vi "FestoCPX.Init.vi"(8 "error in (no error)":errorcluster, 11 "Data in":T1={"Status"={"State"=enum."First", "Conn"=refnum, "TS"=timestamp(0 s since 1904-01-01)}, "Sets"={"IP"="", "Timeout_ms"=1, "ReconnectPeriod_s"=0, "Config.DI"=[], "Config.DO"=[]}}) -> (0 "error out":errorcluster, 3 "Data out":T1={"Status"={"State"=enum."First", "Conn"=refnum, "TS"=timestamp(0 s since 1904-01-01)}, "Sets"={"IP"="", "Timeout_ms"=1, "ReconnectPeriod_s"=0, "Config.DI"=[], "Config.DO"=[]}})   [LabVIEW 2015]
uses:
  FestoCPX.Data.ctl
  FestoCPX.Data.Status.ctl
  FestoCPX.State.ctl
  FestoCPX.Data.Sets.ctl
  FestoCPX.DI.Sets.ctl
  FestoCPX.DI.ctl
  FestoCPX.DO.Sets.ctl
  FestoCPX.DO.ctl
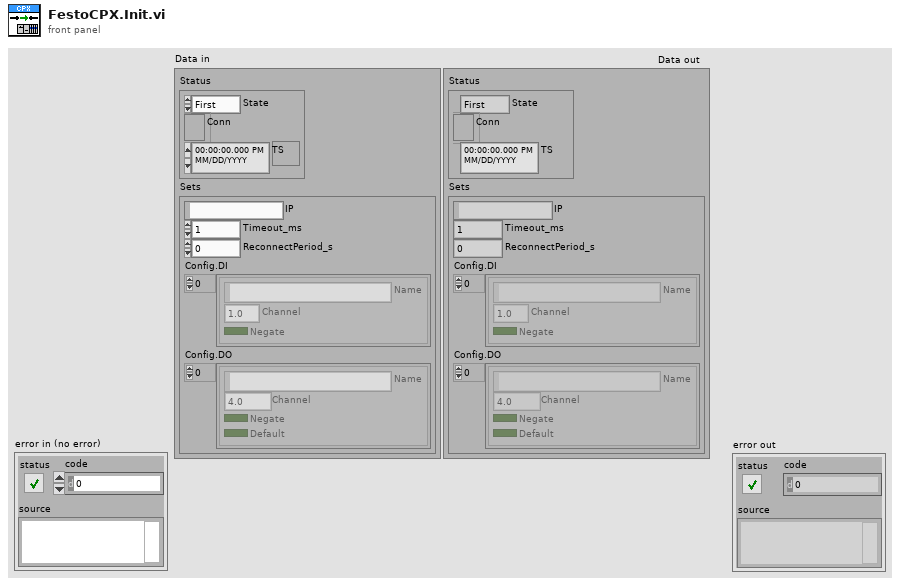
[diagram p1: front panel]
types:
  T1 = typedef "FestoCPX.Data.ctl" = cluster{"Status":T2, "Sets":T4}
  T2 = typedef "FestoCPX.Data.Status.ctl" = cluster{"State":T3, "Conn":refnum<k5>, "TS":timestamp}
  T3 = typedef "FestoCPX.State.ctl" = enum16{"First", "Error", "Init", "Run"}
  T4 = typedef "FestoCPX.Data.Sets.ctl" = cluster{"IP":string, "Timeout_ms":i32, "ReconnectPeriod_s":i32, "Config.DI":T5[], "Config.DO":T7[]}
  T5 = typedef "FestoCPX.DI.Sets.ctl" = cluster{"Name":string, "Channel":T6, "Negate":bool}
  T6 = typedef "FestoCPX.DI.ctl" = enum16{"0.0", "0.1", "0.2", "0.3", "0.4", "0.5", "0.6", "0.7", "1.0", "1.1", "1.2", "1.3", "1.4", "1.5", "1.6", "1.7", "2.0", "2.1", "2.2", "2.3", "2.4", "2.5", "2.6", "2.7", "3.0", "3.1", "3.2", "3.3", "3.4", "3.5", "3.6", "3.7", "4.0", "4.1", "4.2", "4.3", "4.4", "4.5", "4.6", "4.7"}
  T7 = typedef "FestoCPX.DO.Sets.ctl" = cluster{"Name":string, "Channel":T8, "Negate":bool, "Default":bool}
  T8 = typedef "FestoCPX.DO.ctl" = enum16{"4.0", "4.1", "4.2", "4.3", "4.4", "4.5", "4.6", "4.7", "5.0", "5.1", "5.2", "5.3", "5.4", "5.5", "5.6", "5.7", "6.0", "6.1", "6.2", "6.3", "6.4", "6.5", "6.6", "6.7", "Q1K1", "Q1K2", "Q2K1", "Q2K2", "Q3K1", "Q3K2", "Q4K1", "Q4K2", "Q5K1", "Q5K2"}
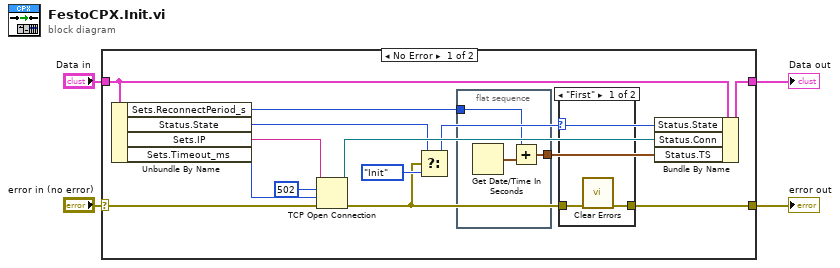
[diagram p0: block diagram]
diagram:
  n1 = case shown="No Error" "error in (no error)" {
    selector: "error in (no error)" -> [w16 w26]
    tunnel: [w12 w26] -> w3
    tunnel: "Data in" -> [w14 w25]
    tunnel: [w18 w25] -> w1
    frame No Error {
      n2 = Unbundle By Name(w14) -> ("Sets.ReconnectPeriod_s"=w6:i32, "Status.State"=w8:T3, "Sets.IP"=w13:string, "Sets.Timeout_ms"=w15:i32)
      n3 = TCP Open Connection(address=w13, remote port or service name=u16 502, timeout ms (60000)=w15, error in (no error)=w16) -> (connection ID=w11:refnum<k5>, error out=w9:errorcluster)  [unwired: 1 in]
      n4 = Select(t=w8, s=w9, f=FestoCPX.State."Init") -> (s? t:f=w7:T3)
      n5 = flat-sequence {
        tunnel: w6 -> [w20]
        tunnel: [w19] -> w5
        frame #0 {
          n6 = Get Date/Time In Seconds() -> (seconds since 1Jan1904=w21:timestamp)
          n7 = Add(x=w20, y=w21) -> (x+y=w19:timestamp)
        }
      }
      n8 = case shown="\"First\"" w7 {
        tunnel: w9 -> [w23 w24]
        tunnel: [w22 w24] -> w12
        frame "First" {
          n9 = call <vilib>:"Clear Errors.vi"("error in (no error)"=w23) -> ("error out"=w22:errorcluster)  [unwired: 5 in, 1 out]
        }
        frame Default {
        }
      }
      n10 = Bundle By Name(cluster=w14, "Status.State"=w7, "Status.Conn"=w11, "Status.TS"=w5) -> (w18:T1)
    }
    frame Error {
    }
  }
  "error out" <- w3
  "Data out" <- w1
